vi "inline_table_set_sub_table_item.vi"(6 "close_item? (true)":bool=TRUE, 7 "subtables":string[](array[string]), 8 "error in (no error)":errorcluster, 9 "item (value)":refnum<class "Item.lvclass">, 10 "key":string, 11 "InlineTable in":refnum<class "InlineTable.lvclass">) -> (0 "error out":errorcluster, 3 "InlineTable out":refnum<class "InlineTable.lvclass">)   [LabVIEW 2020, in "toml.lvclass"]
uses:
  toml.lvclass
  Item/Item.lvclass
  InlineTable/InlineTable.lvclass
  toml.lvclass/toml.ctl
  Value/Value.lvclass
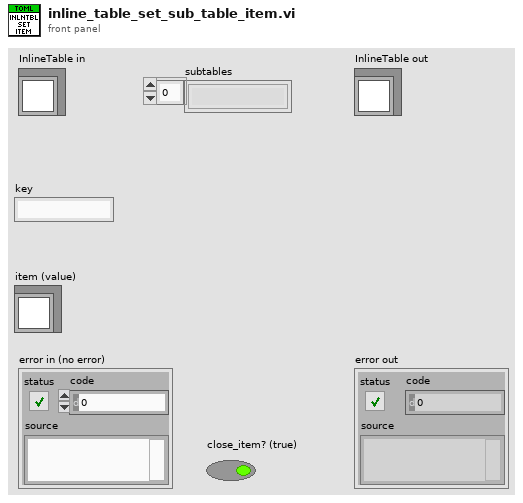
[diagram p1: front panel]
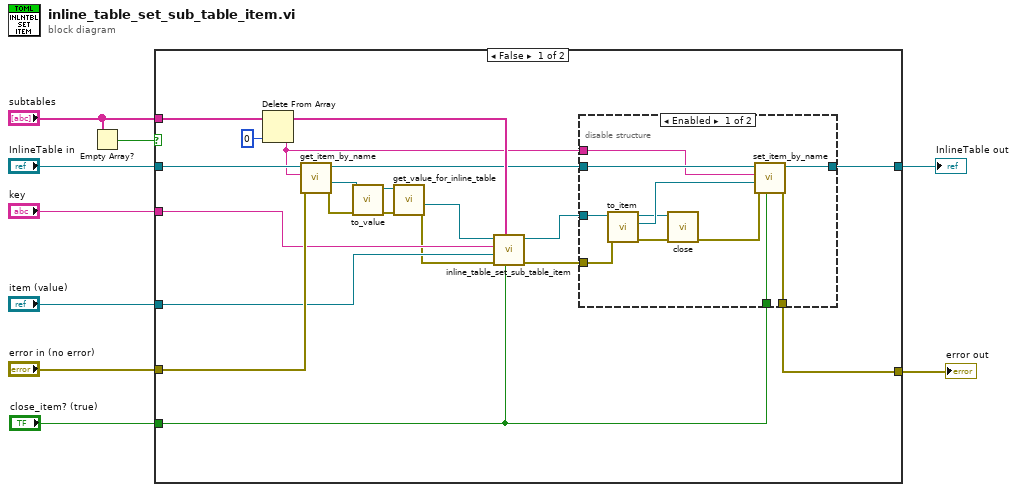
[diagram p0: block diagram]
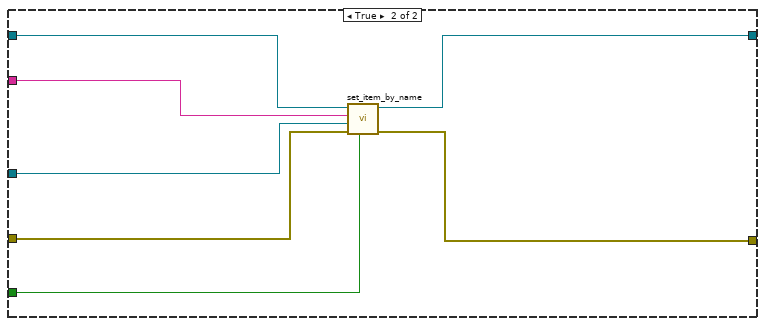
[diagram p3: hidden frame]
diagram:
  n1 = Empty Array?(array="subtables") -> (empty?=w4:bool)
  n2 = case shown="False" w4 {
    tunnel: [w22 w49] -> w9
    tunnel: "item (value)" -> [w23 w46]
    tunnel: [w18 w48] -> w7
    tunnel: "InlineTable in" -> [w26 w47]
    tunnel: "error in (no error)" -> [w25 w45]
    tunnel: "subtables" -> [w29 _]
    tunnel: "close_item? (true)" -> [w10 w44]
    tunnel: "key" -> [w17 w43]
    frame False {
      n3 = Delete From Array(array=w29, index=0) -> (deleted portion=w21:string, array with subset deleted=w27:string[])  [unwired: 1 in]
      n4 = call "get_item_by_name.vi"("error in (no error)"=w25, "key_name"=w21, "Table in"=w26) -> ("error out"=w13:errorcluster, "Item"=w14:refnum<class "Item.lvclass">, "Table out"=w24:refnum<class "InlineTable.lvclass">)  [unwired: 6 in]
      n5 = call "to_value.vi"("error in (no error)"=w13, "Item in"=w14) -> ("error out"=w15:errorcluster, "Value out"=w16:refnum<class "Value.lvclass">)  [unwired: 8 in]
      n6 = call "get_value_for_inline_table.vi"("error in (no error)"=w15, "Value in"=w16) -> ("error out"=w11:errorcluster, "InlineTable out"=w12:refnum<class "InlineTable.lvclass">)  [unwired: 7 in, 1 out]
      n7 = call "inline_table_set_sub_table_item.vi"("close_item? (true)"=w10, "subtables"=w27, "error in (no error)"=w11, "item (value)"=w23, "key"=w17, "InlineTable in"=w12) -> ("error out"=w19:errorcluster, "InlineTable out"=w20:refnum<class "InlineTable.lvclass">)  [unwired: 4 in]
      n8 = disable-structure shown="Enabled" {
        disable-tunnel: w24 -> [w40 w42]
        disable-tunnel: [w39 w41] -> w22
        disable-tunnel: w21 -> [w38 _]
        disable-tunnel: w20 -> [w36 _]
        disable-tunnel: w19 -> [w35 w41]
        disable-tunnel: [w31 w42] -> w18
        disable-tunnel: w10 -> [w30 _]
        frame Enabled {
          n9 = call "to_item.vi"("error in (no error)"=w35, "Table in"=w36) -> ("error out"=w33:errorcluster, "Item out"=w37:refnum<class "Item.lvclass">, "Table out"=w34:refnum<class "InlineTable.lvclass">)  [unwired: 7 in]
          n10 = call "close.vi"("error in (no error)"=w33, "Table in"=w34) -> ("error out"=w32:errorcluster)  [unwired: 9 in]
          n11 = call "set_item_by_name.vi"("close_item? (true)"=w30, "error in"=w32, "Item"=w37, "key_name"=w38, "Table in"=w40) -> ("error out"=w39:errorcluster, "Table out"=w31:refnum<class "InlineTable.lvclass">)  [unwired: 5 in]
        }
        frame Disabled {
        }
      }
    }
    frame True {
      n12 = call "set_item_by_name.vi"("close_item? (true)"=w44, "error in"=w45, "Item"=w46, "key_name"=w43, "Table in"=w47) -> ("error out"=w49:errorcluster, "Table out"=w48:refnum<class "InlineTable.lvclass">)  [unwired: 5 in]
    }
  }
  "error out" <- w9
  "InlineTable out" <- w7
